vi "myrio_testxbeelink.vi"() -> ()   [LabVIEW 2014]
uses:
  <vilib>/myRIO/Instrument Drivers/Onboard IO/DIO/typedefs/DIO Reference.ctl
  <vilib>/myRIO/Common/Instrument Driver Framework/Utilities/typedefs/myRIO Generic Hardware Reference.ctl
  <vilib>/myRIO/Common/Instrument Driver Framework/Utilities/typedefs/Hardware Version Enum.ctl
  <vilib>/myRIO/Common/Instrument Driver Framework/Utilities/typedefs/myRIO v1.0 Reference.ctl
  <vilib>/myRIO/Common/Instrument Driver Framework/Utilities/typedefs/Generic FPGA Reference.ctl
  <vilib>/myRIO/Common/Instrument Driver Framework/myRIO v1.0/DIO/typedefs/DIO Channels List.ctl
  <vilib>/myRIO/Common/Instrument Driver Framework/myRIO v1.0/DIO/typedefs/DIO Channels Enum.ctl
  <vilib>/userdefined/High Color/nirio_resource_hc.ctl
  <vilib>/Instr/_visa.llb/VISA Flush IO Buffer Mask.ctl
  <vilib>/myRIO/Common/Instrument Driver Framework/myRIO v1.0/DIO/vis/myRIO v1.1 Open DIO.vi
  <vilib>/myRIO/Common/Instrument Driver Framework/Utilities/vis/Validate Channels.vi
  <vilib>/myRIO/Common/Instrument Driver Framework/myRIO v1.0/DIO/vis/myRIO v1.0 Reserve DIO.vi
  <vilib>/myRIO/Common/Instrument Driver Framework/myRIO v1.0/DIO/vis/myRIO v1.0 Close DIO.vi
  <vilib>/myRIO/Common/Instrument Driver Framework/myRIO v1.0/Resource Manager/vis/myRIO v1.0 Reserve Channel List.vi
  <vilib>/myRIO/Common/Instrument Driver Framework/myRIO v1.0/DIO/vis/myRIO v1.0 Build MUX Configuration DIO.vi
  <vilib>/myRIO/Common/Instrument Driver Framework/myRIO v1.0/DIO/vis/myRIO v1.0 Unreserve DIO.vi
  <vilib>/myRIO/Common/Instrument Driver Framework/myRIO v1.0/Resource Manager/vis/myRIO v1.0 Reserve Channel.vi
  <vilib>/myRIO/Common/Instrument Driver Framework/myRIO v1.0/Resource Manager/vis/myRIO v1.0 Unreserve Channel.vi
  <vilib>/myRIO/Common/Instrument Driver Framework/myRIO v1.0/Resource Manager/vis/myRIO v1.0 Create Configuration List.vi
  <vilib>/myRIO/Common/Instrument Driver Framework/myRIO v1.0/Resource Manager/vis/myRIO v1.0 Unreserve Channel List.vi
  <vilib>/myRIO/Common/Instrument Driver Framework/myRIO v1.0/Resource Manager/vis/myRIO v1.0 Build Mutex Name.vi
  <vilib>/Utility/VariantDataType/GetNumericInfo.vi
  <vilib>/Utility/error.llb/Error Cluster From Error Code.vi
  <vilib>/myRIO/Common/Instrument Driver Framework/myRIO v1.0/myRIO v1.1 Open.vi
  <vilib>/myRIO/Common/Instrument Driver Framework/Utilities/vis/IO Manager.vi
  <vilib>/myRIO/Common/Instrument Driver Framework/Utilities/vis/Configuration Manager.vi
  <vilib>/myRIO/Common/Instrument Driver Framework/myRIO v1.0/Resource Manager/vis/myRIO v1.0 Configure IO.vi
  <vilib>/myRIO/Common/Instrument Driver Framework/myRIO v1.0/myRIO v1.0 Close.vi
  <vilib>/myRIO/Common/Instrument Driver Framework/myRIO v1.0/DIO/vis/myRIO v1.0 Write DIO.vi
  <vilib>/myRIO/Common/Instrument Driver Framework/myRIO v1.0/DIO/vis/myRIO v1.0 Shutdown DIO.vi
  <vilib>/myRIO/Instrument Drivers/Onboard IO/DIO/vis/myRIO DIO Open.xnode
  <vilib>/myRIO/Instrument Drivers/Onboard IO/DIO/DIO.lvlib
panel:
  in  "Tab Control":T1(tab)
  in  "Communication Link\nVISA Port":refnum<visa-resource-name>="ASRL1::INSTR"
  in  "GPS Link\nVISA Port":refnum<visa-resource-name>="ASRL2::INSTR"
  in  "Communication Link\nError In":errorcluster
  in  "GPS Link\nError In":errorcluster
  out "Handshake Complete?":bool
  out "Handshake Aborted":bool
  out "Comms Network \nHandshake Successful?":bool
  out "GPS Network \nHandshake Successful?":bool
  out "Comms String":string
  out "GPS String":string
  out "LED Error Out":errorcluster
  out "Running?":bool
  in  "[ESC]":bool
  out "error out":errorcluster
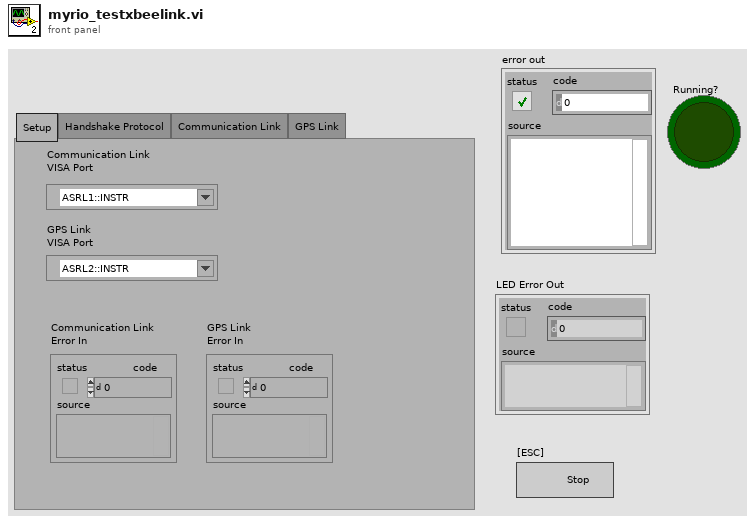
[diagram p1: front panel]
types:
  T1 = enum32{"Setup", "Handshake Protocol", "Communication Link", "GPS Link"}
  T2 = typedef "nirio_resource_hc.ctl" = tag
  T3 = typedef "Hardware Version Enum.ctl" = enum16{"Unknown", "myRIO-1900", "myRIO-1950"}
  T4 = typedef "DIO.lvlib/DIO Reference.ctl" = cluster{"myRIO Reference":T5, "DIO Channels List":T8}
  T5 = typedef "myRIO Generic Hardware Reference.ctl" = cluster{"myRIO Model":T3, "myRIO Hardware Reference":T6}
  T6 = typedef "myRIO v1.0 Reference.ctl" = cluster{"Generic FPGA Reference":T7, "Allow multiple opens":bool}
  T7 = typedef "Generic FPGA Reference.ctl" = refnum<k20>
  T8 = typedef "DIO Channels List.ctl" = T9[]
  T9 = typedef "DIO Channels Enum.ctl" = enum16{"Not Connected", "C/DIO0", "C/DIO1", "C/DIO2", "C/DIO3", "C/DIO4", "C/DIO5", "C/DIO6", "C/DIO7", "A/DIO0", "A/DIO1", "A/DIO2", "A/DIO3", "A/DIO4", "A/DIO5", "A/DIO6", "A/DIO7", "A/DIO8", "A/DIO9", "A/DIO10", "A/DIO11", "A/DIO12", "A/DIO13", "A/DIO14", "A/DIO15", "B/DIO0", "B/DIO1", "B/DIO2", "B/DIO3", "B/DIO4", "B/DIO5", "B/DIO6", "B/DIO7", "B/DIO8", "B/DIO9", "B/DIO10", "B/DIO11", "B/DIO12", "B/DIO13", "B/DIO14", "B/DIO15", "LED0", "LED1", "LED2", "LED3", "Button0"}
  T10 = typedef "VISA Flush IO Buffer Mask.ctl" = u16
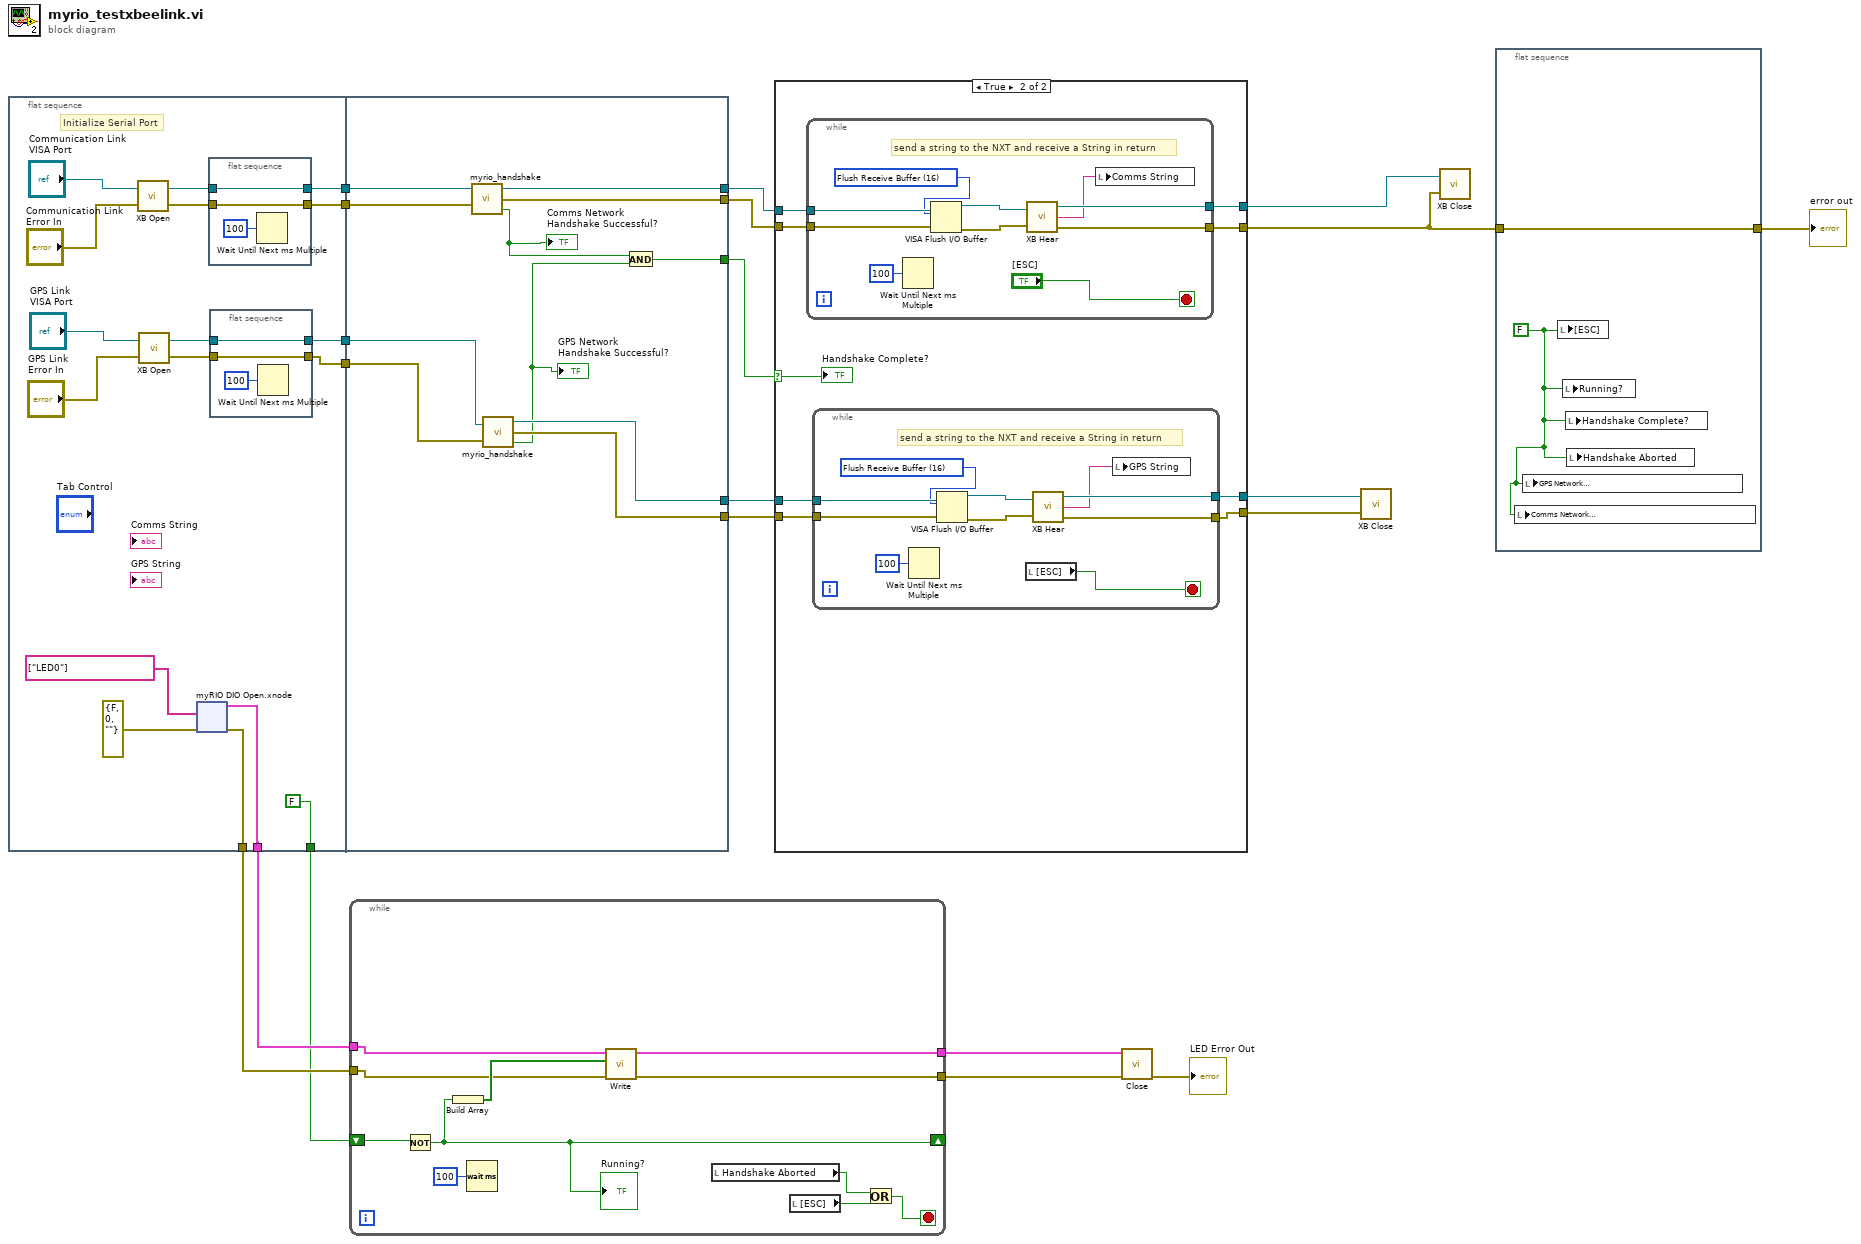
[diagram p0: block diagram]
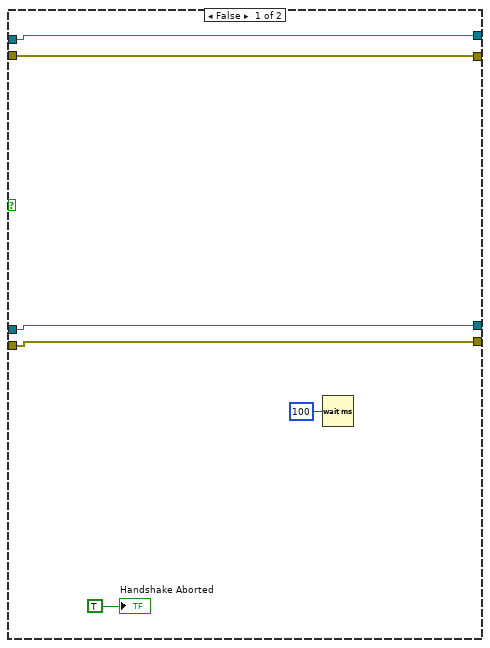
[diagram p2: hidden frame]
diagram:
  n1 = flat-sequence {
    tunnel: [w33] -> w16
    tunnel: [w32] -> w15
    tunnel: [w29] -> w13
    tunnel: [w28] -> w14
    tunnel: [FALSE] -> w12
    tunnel: [w22] -> w7
    tunnel: [w21] -> w6
    tunnel: w16 -> [w70]
    tunnel: w15 -> [w69]
    tunnel: [w68] -> w9
    tunnel: [w67] -> w8
    tunnel: w7 -> [w66]
    tunnel: w6 -> [w65]
    tunnel: [w64] -> w4
    tunnel: [w63] -> w3
    tunnel: [w62] -> w5
    frame #0 {
      # "Initialize Serial Port"
      n2 = call "XB Open.vi"("error in (no error)"="Communication Link\nError In", "VISA resource name"="Communication Link\nVISA Port") -> ("error out"=w36:errorcluster, "VISA resource name out"=w37:refnum<visa-resource-name>)
      n3 = call "XB Open.vi"("error in (no error)"="GPS Link\nError In", "VISA resource name"="GPS Link\nVISA Port") -> ("error out"=w24:errorcluster, "VISA resource name out"=w23:refnum<visa-resource-name>)
      n4 = xnode "myRIO DIO Open.xnode"("error in (no error)"=errorcluster {"status"=FALSE, "code"=0, "source"=""}, "Channel Names"=tag[] ["LED0"]) -> ("error out"=w28:errorcluster, "DIO Ref Out"=w29:T4)  [unwired: 1 in]
      n5 = flat-sequence {
        tunnel: w37 -> [w57]
        tunnel: w36 -> [w58]
        tunnel: [w58] -> w32
        tunnel: [w57] -> w33
        frame #0 {
          n6 = Wait Until Next ms Multiple(millisecond multiple=u32 100) -> ()  [unwired: 1 out]
        }
      }
      n7 = flat-sequence {
        tunnel: w23 -> [w38]
        tunnel: w24 -> [w39]
        tunnel: [w39] -> w21
        tunnel: [w38] -> w22
        frame #0 {
          n8 = Wait Until Next ms Multiple(millisecond multiple=u32 100) -> ()  [unwired: 1 out]
        }
      }
    }
    frame #1 {
      n9 = call "myrio_handshake.vi"("VISA resource name"=w70, "error in"=w69) -> ("VISA resource name out"=w68:refnum<visa-resource-name>, "error out"=w67:errorcluster, "All Clear \nfrom PC?"=w61:bool)
      "Comms Network \nHandshake Successful?" <- w61
      n10 = call "myrio_handshake.vi"("VISA resource name"=w66, "error in"=w65) -> ("VISA resource name out"=w64:refnum<visa-resource-name>, "error out"=w63:errorcluster, "All Clear \nfrom PC?"=w60:bool)
      "GPS Network \nHandshake Successful?" <- w60
      n11 = And(x=w61, y=w60) -> (x .and. y?=w62:bool)
    }
  }
  n12 = while {
    tunnel: w13 -> [w78]
    tunnel: w14 -> [w77]
    shift-right: [w74] -> _
    shift-left: w12 -> [w80]
    tunnel: [w76] -> w19
    tunnel: [w75] -> w18
    stop <- w72 stop-if-true
    n13 = Not(x=w80) -> (.not. x?=w74:bool)
    "Running?" <- w74
    n14 = Build Array(w74) -> (w79:bool[])
    n15 = Wait (ms)(milliseconds to wait=u32 100) -> ()  [unwired: 1 out]
    n16 = call <vilib>:"Write.vi"("error in (no error)"=w77, "Values"=w79, "DIO Ref In"=w78) -> ("error out"=w76:errorcluster, "DIO Ref Out"=w75:T4)  [unwired: 6 in]
    n17 = local read "Handshake Aborted"() -> (w71:bool)
    n18 = local read "[ESC]"() -> (w73:bool)
    n19 = Or(x=w71, y=w73) -> (x .or. y?=w72:bool)
  }
  n20 = case shown="True" w5 {
    selector: w5 -> [_ w92]
    tunnel: [w86 w96] -> w20
    tunnel: w9 -> [w86 w95]
    tunnel: w8 -> [w87 w94]
    tunnel: [w87 w93] -> w10
    tunnel: w4 -> [w83 w91]
    tunnel: w3 -> [w82 w90]
    tunnel: [w83 w89] -> w2
    tunnel: [w82 w88] -> w1
    frame False {
      n21 = Wait (ms)(milliseconds to wait=u32 100) -> ()  [unwired: 1 out]
      "Handshake Aborted" <- TRUE
    }
    frame True {
      n22 = while {
        tunnel: w95 -> [w111]
        tunnel: [w116] -> w93
        tunnel: [w115] -> w96
        tunnel: w94 -> [w107]
        stop <- "[ESC]" stop-if-true
        w109 = T10 16 items=["Flush Receive Buffer"=16, "Write Transmit Buffer to Device"=32, "Flush Receive Buffer (No I/O)"=64, "Flush Transmit Buffer"=128] ("Mask")
        # "send a string to the NXT and receive a String in return"
        n23 = Wait Until Next ms Multiple(millisecond multiple=u32 100) -> ()  [unwired: 1 out]
        n24 = VISA Flush I/O Buffer(VISA resource name=w111, mask (16)=w109, error in (no error)=w107) -> (VISA resource name out=w110:refnum<visa-resource-name>, error out=w112:errorcluster)
        n25 = call "XB Hear.vi"("VISA resource name"=w110, "error in (no error)"=w112) -> ("VISA resource name out"=w115:refnum<visa-resource-name>, "String Received"=w113:string, "error out"=w116:errorcluster)
        n26 = local write "Comms String"(w113) -> ()
      }
      n27 = while {
        tunnel: w91 -> [w101]
        tunnel: [w106] -> w88
        tunnel: [w105] -> w89
        tunnel: w90 -> [w98]
        stop <- w97 stop-if-true
        w99 = T10 16 items=["Flush Receive Buffer"=16, "Write Transmit Buffer to Device"=32, "Flush Receive Buffer (No I/O)"=64, "Flush Transmit Buffer"=128] ("Mask")
        # "send a string to the NXT and receive a String in return"
        n28 = Wait Until Next ms Multiple(millisecond multiple=u32 100) -> ()  [unwired: 1 out]
        n29 = VISA Flush I/O Buffer(VISA resource name=w101, mask (16)=w99, error in (no error)=w98) -> (VISA resource name out=w100:refnum<visa-resource-name>, error out=w102:errorcluster)
        n30 = local read "[ESC]"() -> (w97:bool)
        n31 = call "XB Hear.vi"("VISA resource name"=w100, "error in (no error)"=w102) -> ("VISA resource name out"=w105:refnum<visa-resource-name>, "String Received"=w103:string, "error out"=w106:errorcluster)
        n32 = local write "GPS String"(w103) -> ()
      }
      "Handshake Complete?" <- w92
    }
  }
  n33 = call <vilib>:"Close.vi"("error in (no error)"=w19, "DIO Ref In"=w18) -> ("error out"=→"LED Error Out":errorcluster)  [unwired: 9 in]
  n34 = call "XB Close.vi"("error in (no error)"=w1, "VISA resource name"=w2) -> ()
  n35 = call "XB Close.vi"("error in (no error)"=w10, "VISA resource name"=w20) -> ()
  n36 = flat-sequence {
    tunnel: [w118] -> w11
    tunnel: w10 -> [w118]
    frame #0 {
      w117 = FALSE
      n37 = local write "Comms Network \nHandshake Successful?"(w117) -> ()
      n38 = local write "GPS Network \nHandshake Successful?"(w117) -> ()
      n39 = local write "[ESC]"(w117) -> ()
      n40 = local write "Running?"(w117) -> ()
      n41 = local write "Handshake Complete?"(w117) -> ()
      n42 = local write "Handshake Aborted"(w117) -> ()
    }
  }
  "error out" <- w11
